vi "CMD_Sanic.vi"(1 "Line":string) -> (0 "Done":bool)   [LabVIEW 2014]
panel:
  in  "Parameters":i32[](array[numeric])=[1, 3, 1, 3, 1]
  in  "Subcommands":string[](array[string])=["at", "at", "for", "to", "until"]
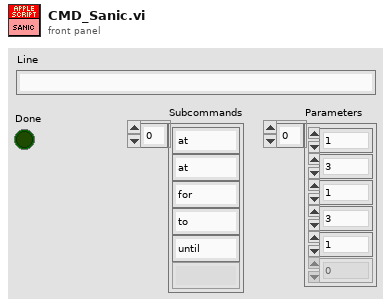
[diagram p1: front panel]
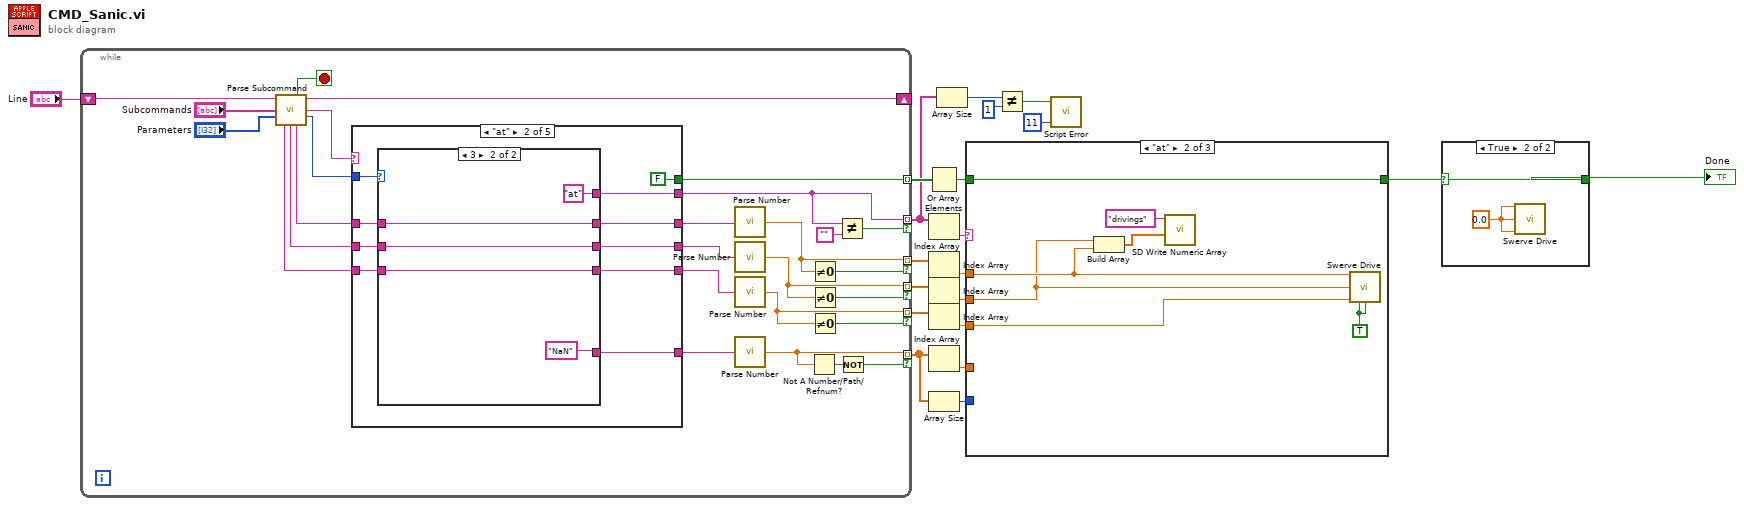
[diagram p0: block diagram]
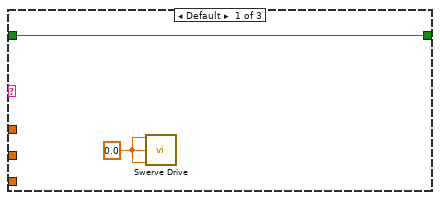
[diagram p3: hidden frame]
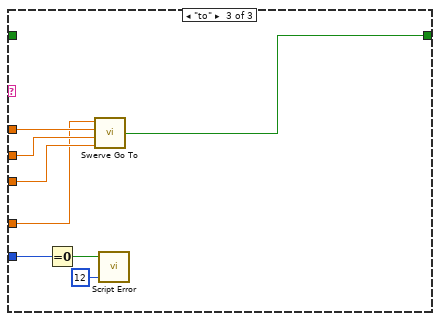
[diagram p4: hidden frame]
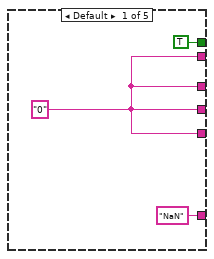
[diagram p5: hidden frame]
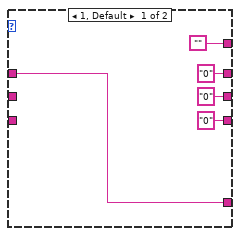
[diagram p6: hidden frame]
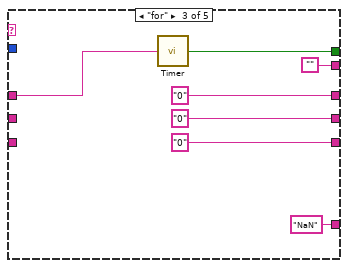
[diagram p7: hidden frame]
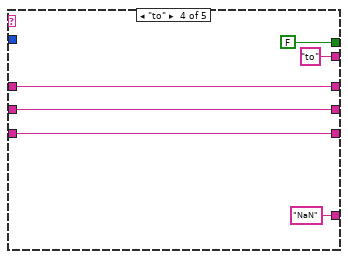
[diagram p8: hidden frame]
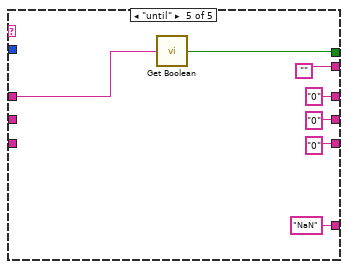
[diagram p9: hidden frame]
diagram:
  n1 = while {
    shift-right: [w44] -> _
    shift-left: "Line" -> [w47]
    tunnel: [w21] -> w5 mode=indexing
    tunnel: [w33] -> w17 mode=indexing if=w27
    tunnel: [w32] -> w15 mode=indexing if=w25
    tunnel: [w29] -> w13 mode=indexing if=w26
    tunnel: [w24] -> w3 mode=indexing if=w22
    tunnel: [w35] -> w4 mode=indexing if=w36
    stop <- w43 stop-if-true
    n2 = call "Parse Subcommand.vi"("Text In"=w47, "Subcommands"="Subcommands", "Parameters"="Parameters") -> ("Done"=w43:bool, "Text Out"=w44:string, "Subcommand"=w42:string, "# of Parameters"=w41:i32, "Parameter 3"=w39:string, "Parameter 2"=w38:string, "Parameter 1"=w40:string)  [unwired: 6 in]
    n3 = case shown="\"at\"" w42 {
      tunnel: w41 -> [_ w60 _ _ _]
      tunnel: w40 -> [_ w59 w71 w83 w85]
      tunnel: w38 -> [_ w58 _ w82 _]
      tunnel: w39 -> [_ w57 _ w81 _]
      tunnel: [w49 w56 "0" ("Parameter 1") w83 "0" ("Parameter 1")] -> w34
      tunnel: [w49 w55 "0" ("Parameter 2") w82 "0" ("Parameter 1")] -> w31
      tunnel: [w49 w54 "0" ("Parameter 3") w81 "0" ("Parameter 1")] -> w30
      tunnel: [TRUE ("Value") FALSE ("Running") w72 FALSE w84] -> w21
      tunnel: [w49 w51 "" "to" ("format string") ""] -> w35
      tunnel: ["NaN" ("Parameter 1") w53 "NaN" ("Parameter 3") "NaN" ("Parameter 3") "NaN" ("Parameter 1")] -> w28
      frame Default {
        w49 = "0" ("format string")
      }
      frame "at" {
        n4 = case shown="3" w60 {
          tunnel: w59 -> [w63 w70]
          tunnel: w58 -> [_ w69]
          tunnel: w57 -> [_ w66]
          tunnel: ["0" ("Parameter 2") w70] -> w56
          tunnel: ["0" ("Parameter 2") w69] -> w55
          tunnel: ["0" ("Parameter 3") w66] -> w54
          tunnel: [w63 "NaN" ("Parameter 3")] -> w53
          tunnel: ["" "at"] -> w51
          frame 1, Default {
          }
          frame 3 {
          }
        }
      }
      frame "for" {
        n5 = call "Timer.vi"("Seconds (string)"=w71) -> ("Done"=w72:bool)
      }
      frame "to" {
      }
      frame "until" {
        n6 = call "Get Boolean.vi"("Name"=w85) -> ("Value"=w84:bool)
      }
    }
    n7 = call "Parse Number.vi"("String"=w34) -> ("Number"=w33:dbl)
    n8 = call "Parse Number.vi"("String"=w31) -> ("Number"=w32:dbl)
    n9 = call "Parse Number.vi"("String"=w30) -> ("Number"=w29:dbl)
    n10 = call "Parse Number.vi"("String"=w28) -> ("Number"=w24:dbl)
    n11 = Not A Number/Path/Refnum?(number/path/refnum=w24) -> (NaN/Path/Refnum?=w23:bool)
    n12 = Not Equal To 0?(x=w33) -> (x != 0?=w27:bool)
    n13 = Not Equal To 0?(x=w32) -> (x != 0?=w25:bool)
    n14 = Not Equal To 0?(x=w29) -> (x != 0?=w26:bool)
    n15 = Not Equal?(x=w35, y="") -> (x != y?=w36:bool)
    n16 = Not(x=w23) -> (.not. x?=w22:bool)
  }
  n17 = Or Array Elements(Boolean array=w5) -> (logical OR=w1:bool)
  n18 = Index Array(array=w4) -> (element=w10:string)  [unwired: 1 in]
  n19 = Index Array(array=w17) -> (element=w16:dbl)  [unwired: 1 in]
  n20 = Index Array(array=w15) -> (element=w14:dbl)  [unwired: 1 in]
  n21 = Index Array(array=w13) -> (element=w12:dbl)  [unwired: 1 in]
  n22 = Index Array(array=w3) -> (element=w11:dbl)  [unwired: 1 in]
  n23 = Array Size(array=w3) -> (size(s)=w2:i32)
  n24 = Array Size(array=w4) -> (size(s)=w8:i32)
  n25 = case shown="\"at\"" w10 {
    tunnel: w16 -> [_ w97 w107]
    tunnel: w1 -> [w92 w99 _]
    tunnel: [w92 w99 w100] -> w18
    tunnel: w14 -> [_ w96 w106]
    tunnel: w12 -> [_ w93 w105]
    tunnel: w11 -> [_ _ w104]
    tunnel: w2 -> [_ _ w102]
    frame Default {
      w91 = 0.0 ("X")
      n26 = call "Swerve Drive.vi"("X"=w91, "Y"=w91, "Z"=w91) -> ()  [unwired: 13 in]
    }
    frame "at" {
      w94 = TRUE ("Auto Controls")
      n27 = Build Array(w96, w97) -> (w95:dbl[])
      n28 = call <vilib>:"SD Write Numeric Array.vi"("Numeric Array"=w95, "Name"="drivings") -> ()  [unwired: 8 in, 2 out]
      n29 = call "Swerve Drive.vi"("X"=w97, "Y"=w96, "Z"=w93, "Auto Controls"=w94, "Robot-Centric"=w94) -> ()  [unwired: 11 in]
    }
    frame "to" {
      n30 = Equal To 0?(x=w102) -> (x = 0?=w101:bool)
      n31 = call "Swerve Go To.vi"("Max Speed"=w104, "Target X"=w107, "Target Y"=w106, "Target Angle"=w105) -> ("Done"=w100:bool)  [unwired: 3 in]
      n32 = call "Script Error.vi"("Error?"=w101, "Error Code"=12) -> ()  [unwired: 3 in, 1 out]
    }
  }
  n33 = Not Equal?(x=w8, y=1) -> (x != y?=w6:bool)
  n34 = call "Script Error.vi"("Error?"=w6, "Error Code"=11) -> ()  [unwired: 3 in, 1 out]
  n35 = case shown="True" w18 {
    selector: w18 -> [w108 w110]
    tunnel: [w108 w110] -> w19
    frame False {
    }
    frame True {
      w109 = 0.0 ("X")
      n36 = call "Swerve Drive.vi"("X"=w109, "Y"=w109, "Z"=w109) -> ()  [unwired: 13 in]
    }
  }
  "Done" <- w19
